vi "Size.vi"(7 "DPI":dbl=nan, 8 "error in (no error)":errorcluster, 9 "Height (pixels)":dbl=nan, 10 "Width (pixels)":dbl=nan, 11 "Plot ID":T1 format="%x") -> (0 "error out":errorcluster, 3 "Plot ID Out":T1 format="%x")   [LabVIEW 2013, in "Advanced Plotting Toolkit.lvlib"]
doc: "Resize a plot. Width, height, and DPI inputs are all optiona.\n\nPlots are stored interally as vector art, and may be repeatedly resized without loss of detail. The DPI (dots-per-inch) is used for conversion between pixels and inches, and when saving as PDF.\n\nNew plots are 640x480, with a DPI of 80."
uses:
  Advanced Plotting Toolkit.lvlib
  typedefs/PlotID.ctl
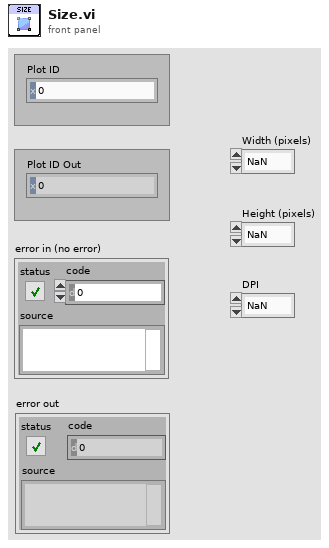
[diagram p1: front panel]
types:
  T1 = typedef "Advanced Plotting Toolkit.lvlib/PlotID.ctl" = i32
  T2 = typedef "Advanced Plotting Toolkit.lvlib/KeyValue.ctl" = cluster{"Key":string, "Value":string}
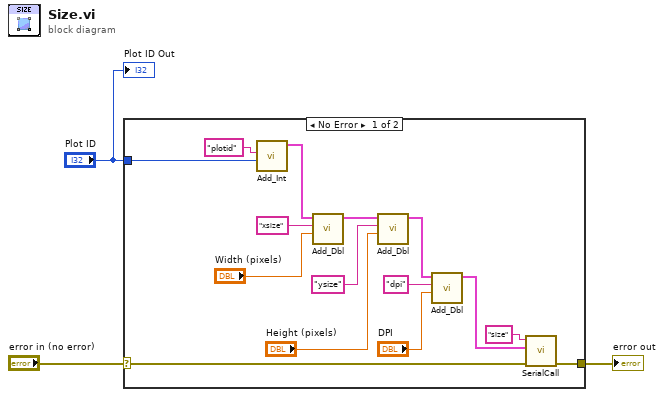
[diagram p0: block diagram]
diagram:
  n1 = case shown="No Error" "error in (no error)" {
    selector: "error in (no error)" -> [w10 w19]
    tunnel: "Plot ID" -> [w9 _]
    tunnel: [w4 w19] -> w2
    frame No Error {
      n2 = call "Add_Int.vi"("Value"=w9, "Key"="plotid") -> ("Keyword Array Out"=w5:T2[])  [unwired: 9 in]
      n3 = call "Add_Dbl.vi"("Value"="Width (pixels)", "Key"="xsize", "Keyword Array"=w5) -> ("Keyword Array Out"=w14:T2[])  [unwired: 8 in]
      n4 = call "Add_Dbl.vi"("Value"="Height (pixels)", "Key"="ysize", "Keyword Array"=w14) -> ("Keyword Array Out"=w13:T2[])  [unwired: 8 in]
      n5 = call "Add_Dbl.vi"("Value"="DPI", "Key"="dpi", "Keyword Array"=w13) -> ("Keyword Array Out"=w12:T2[])  [unwired: 8 in]
      n6 = call "SerialCall.vi"("error in (no error)"=w10, "data"=w12, "Resource"="size") -> ("error out"=w4:errorcluster)  [unwired: 7 in, 1 out]
    }
    frame Error {
    }
  }
  "error out" <- w2
  "Plot ID Out" <- "Plot ID"
